vi "Error Name.vi"(9 "Signal":bool[](array[boolean]), 11 "Error Name":string[](array[string])=["Key Paid1(AI0)", "Key Paid1(AI1)", "Key Paid1(AI09)", "Key Paid1(AI10)", "Key Paid1(AI11)", "Key Paid1(AI12)"]) -> (3 "Error Message":string)   [LabVIEW 2015]
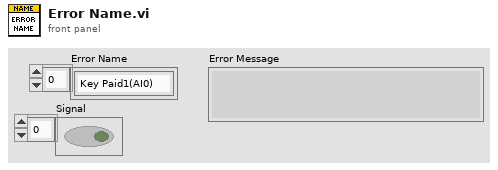
[diagram p1: front panel]
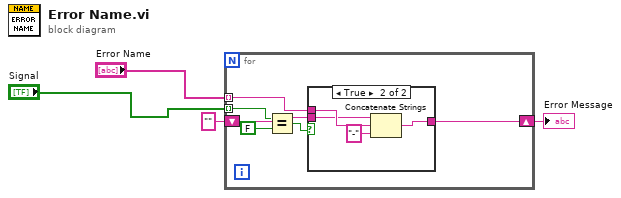
[diagram p0: block diagram]
diagram:
  n1 = for {
    tunnel: "Error Name" -> [w9] mode=indexing
    shift-right: [w8] -> w4
    shift-left: "" -> [w7]
    tunnel: "Signal" -> [w6] mode=indexing
    n2 = Equal?(x=w6, y=FALSE) -> (x = y?=w5:bool)
    n3 = case shown="True" w5 {
      tunnel: w9 -> [_ w15]
      tunnel: [w11 w14] -> w8
      tunnel: w7 -> [w11 w13]
      frame False {
      }
      frame True {
        n4 = Concatenate Strings(w13, w15, "-" ("string")) -> (w14:string)
      }
    }
  }
  "Error Message" <- w4
